vi "New Client.vi"(8 "error in":errorcluster, 10 "Address":string="ws://localhost:8080/", 11 "Realm":string="default_realm") -> (0 "error out":errorcluster, 3 "WAMP client out":refnum<class "WAMP Client.lvclass">)   [LabVIEW 2021, in "wamplv.lvlib" / "WAMP Client.lvclass"]
uses:
  WAMP Client.lvclass
  <vilib>/LabVIEW Open Source Project/OpenURI/uri/URI.lvclass/URI.ctl
  Private/Comm Handlers/RawSocket TCP Handler/RawSocket TCP Handler.lvclass
  D:/Git/wamplv/Private/Comm Handlers/TCPSocketBasedCommHandlerBase/TCPSocketBasedCommHandlerBase.lvclass
  API/TypeDefs/Transport Type.ctl
  Private/Comm Handlers/Websocket Handler/Websocket Handler.lvclass
  WAMP Client.lvclass/WAMP Client.ctl
  Private/Comm Handlers/TCPSocketBasedCommHandlerBase/TCPSocketBasedCommHandlerBase.lvclass
  D:/Git/wamplv/Private/Comm Handlers/ICommHandler/ICommHandler.lvclass
  <vilib>/Utility/error.llb/Error Cluster From Error Code.vi
  <vilib>/ErrorRing/Error Ring.xnode
  <vilib>/LabVIEW Open Source Project/OpenURI/uri/URI.lvclass
  D:/Git/wamplv/Private/Comm Handlers/CommHandlerBase/CommHandlerBase.lvclass
  D:/Git/wamplv/Private/Comm Handlers/RawSocket TCP Handler/RawSocket TCP Handler.lvclass
  D:/Git/wamplv/Private/Comm Handlers/Websocket Handler/Websocket Handler.lvclass
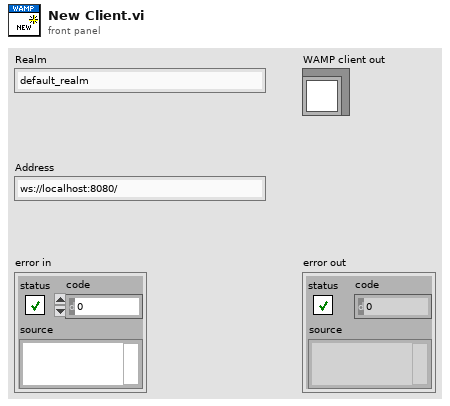
[diagram p1: front panel]
types:
  T1 = typedef "wamplv.lvlib/WAMP Client.lvclass/Transport Type.ctl" = enum16{"WebSocket", "RawSocket TCP"}
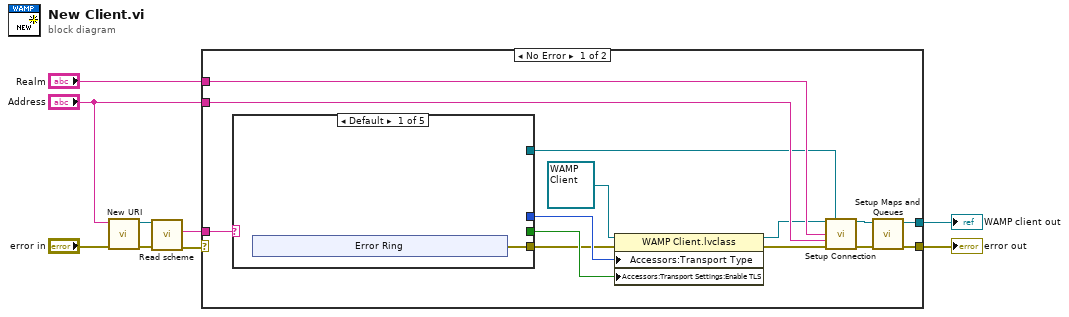
[diagram p0: block diagram]
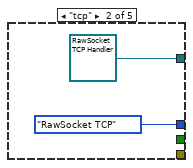
[diagram p2: hidden frame]
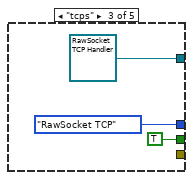
[diagram p3: hidden frame]
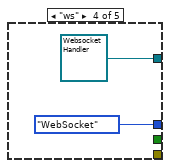
[diagram p4: hidden frame]
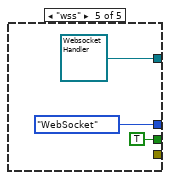
[diagram p5: hidden frame]
diagram:
  n1 = call <vilib>:"New URI.vi"("error in (no error)"="error in", "URI"="Address") -> ("error out"=w4:errorcluster, "URI"=w5:refnum<class "URI.lvclass">)  [unwired: 8 in]
  n2 = call <vilib>:"Read scheme.vi"("error in (no error)"=w4, "URI in"=w5) -> ("error out"=w3:errorcluster, "scheme"=w2:string)  [unwired: 7 in, 1 out]
  n3 = case shown="No Error" w3 {
    selector: w3 -> [_ w39]
    tunnel: "Realm" -> [w23 _]
    tunnel: [w22 _] -> w1
    tunnel: [w21 w39] -> w7
    tunnel: "Address" -> [w20 _]
    tunnel: w2 -> [w19 _]
    frame No Error {
      n4 = case shown="Default" w19 {
        tunnel: [_ refnum<class "RawSocket TCP Handler.lvclass"> refnum ("wamplv.lvlib:RawSocket Handler.lvclass") refnum<class "RawSocket TCP Handler.lvclass"> refnum ("wamplv.lvlib:RawSocket Handler.lvclass") refnum<class "Websocket Handler.lvclass"> refnum ("Websocket Handler.lvclass") refnum<class "Websocket Handler.lvclass"> refnum ("Websocket Handler.lvclass")] -> w18
        tunnel: [w24 _ _ _ _] -> w11
        tunnel: [_ Transport_Type."RawSocket TCP" ("Transport Type") Transport_Type."RawSocket TCP" ("Transport Type") Transport_Type."WebSocket" ("Transport Type") Transport_Type."WebSocket" ("Transport Type")] -> w13
        tunnel: [_ _ TRUE ("Transport Options.Enable TLS?") _ TRUE ("Transport Options.Enable TLS?")] -> w12
        frame Default {
          n5 = xnode "Error Ring"() -> ("error out"=w24:errorcluster)
        }
        frame "tcp" {
        }
        frame "tcps" {
        }
        frame "ws" {
        }
        frame "wss" {
        }
      }
      n6 = property class="WAMP Client.lvclass"(reference=refnum<class "WAMP Client.lvclass"> refnum ("WAMP Client.lvclass"), error in=w11, "Accessors:Transport Type "=w13, "Accessors:Transport Settings:Enable TLS"=w12) -> (reference out=w14:refnum<class "WAMP Client.lvclass">, error out=w10:errorcluster)
      n7 = call-dynamic "Setup Connection.vi"("WAMP Client in"=w14, "ICommHandler.lvclass"=w18, "Realm"=w23, "Address"=w20, "error in (no error)"=w10) -> ("WAMP Client out"=w17:refnum<class "WAMP Client.lvclass">, "error out"=w16:errorcluster)  [unwired: 9 in]
      n8 = call-dynamic "Setup Maps and Queues.vi"("error in (no error)"=w16, "WAMP Client in"=w17) -> ("error out"=w21:errorcluster, "WAMP Client out"=w22:refnum<class "WAMP Client.lvclass">)  [unwired: 8 in]
    }
    frame Error {
    }
  }
  "error out" <- w7
  "WAMP client out" <- w1
